vi "Create directory.vi"(8 "error in (no error)":errorcluster, 10 "Directory":string, 11 "SCP File Transfer in":refnum<class "SCP File Transfer.lvclass">) -> (0 "error out":errorcluster, 3 "SCP File Transfer out":refnum<class "SCP File Transfer.lvclass">)   [LabVIEW 2013, in "PL Framework Configuration Tool.lvlib" / "SCP File Transfer.lvclass"]
doc: "Creates the \"Directory\" on the remote target. The VI also creates all needed directories if the \"Directory\" path contains directories that don't exist on the target.\n\nThe recommended file path format for \"Remote path\" is \"/directory1/directory2\". However, the VI will accept other formats and transform the path appropriately in most cases. Use the \"Strip path.vi\" and \"Build path.vi\" VIs to help with handling remote path strings."
uses:
  SCP File Transfer.lvclass
  <vilib>/NI/RT Management/classes/File Transfer Behavior/File Transfer Behavior.lvclass
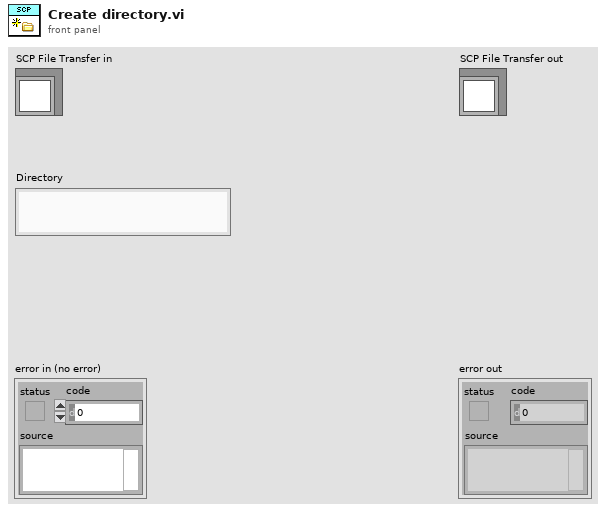
[diagram p1: front panel]
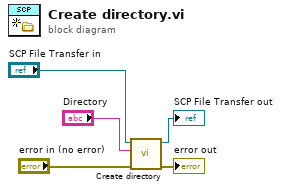
[diagram p0: block diagram]
diagram:
  n1 = call-parent "Create directory.vi"("error in (no error)"="error in (no error)", "Directory"="Directory", "File Transfer Behavior in"="SCP File Transfer in") -> ("error out"=→"error out":errorcluster, "File Transfer Behavior out"=→"SCP File Transfer out":refnum<class "SCP File Transfer.lvclass">)  [unwired: 7 in]
